vi "- VI Tree - JKI SMO.vi"() -> ()   [LabVIEW 2013, in "JKI SMO.lvclass"]
uses:
  JKI SMO.lvclass
  Typedefs/PrivateData--Cluster.ctl
  Typedefs/ProtectedEvents--Cluster.ctl
  Typedefs/StopProcessEventData--Cluster.ctl
  Typedefs/AbortProcessEventData--Cluster.ctl
  Typedefs/RegisteredProcessData--Cluster.ctl
panel:
  in  "JKI SMO.lvclass":refnum<class "JKI SMO.lvclass">
  in  "Process Data":T1
  out "Protected Events":T2
  in  "Abort Processes Event Data":T3
  in  "Stop Processes Event Data":T4
  in  "Private Data":T5
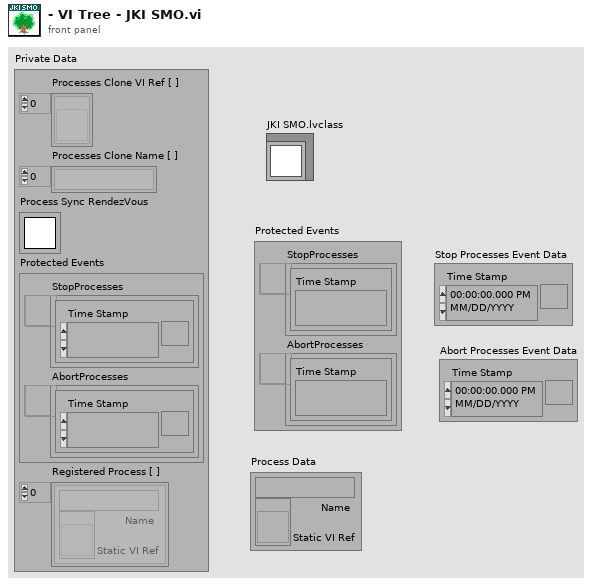
[diagram p1: front panel]
types:
  T1 = typedef "JKI SMO.lvclass/RegisteredProcessData--Cluster.ctl" = cluster{"Name":string, "Static VI Ref":refnum<vi>}
  T2 = typedef "JKI SMO.lvclass/ProtectedEvents--Cluster.ctl" = cluster{"StopProcesses":refnum<user-event>, "AbortProcesses":refnum<user-event>}
  T3 = typedef "JKI SMO.lvclass/AbortProcessEventData--Cluster.ctl" = cluster{"Time Stamp":timestamp}
  T4 = typedef "JKI SMO.lvclass/StopProcessEventData--Cluster.ctl" = cluster{"Time Stamp":timestamp}
  T5 = typedef "JKI SMO.lvclass/PrivateData--Cluster.ctl" = cluster{"Processes Clone VI Ref [ ]":refnum<vi>[], "Processes Clone Name [ ]":string[], "Process Sync RendezVous":T6, "Protected Events":T2, "Registered Process [ ]":T1[]}
  T6 = typedef "Rendezvous RefNum" = refnum<k1>
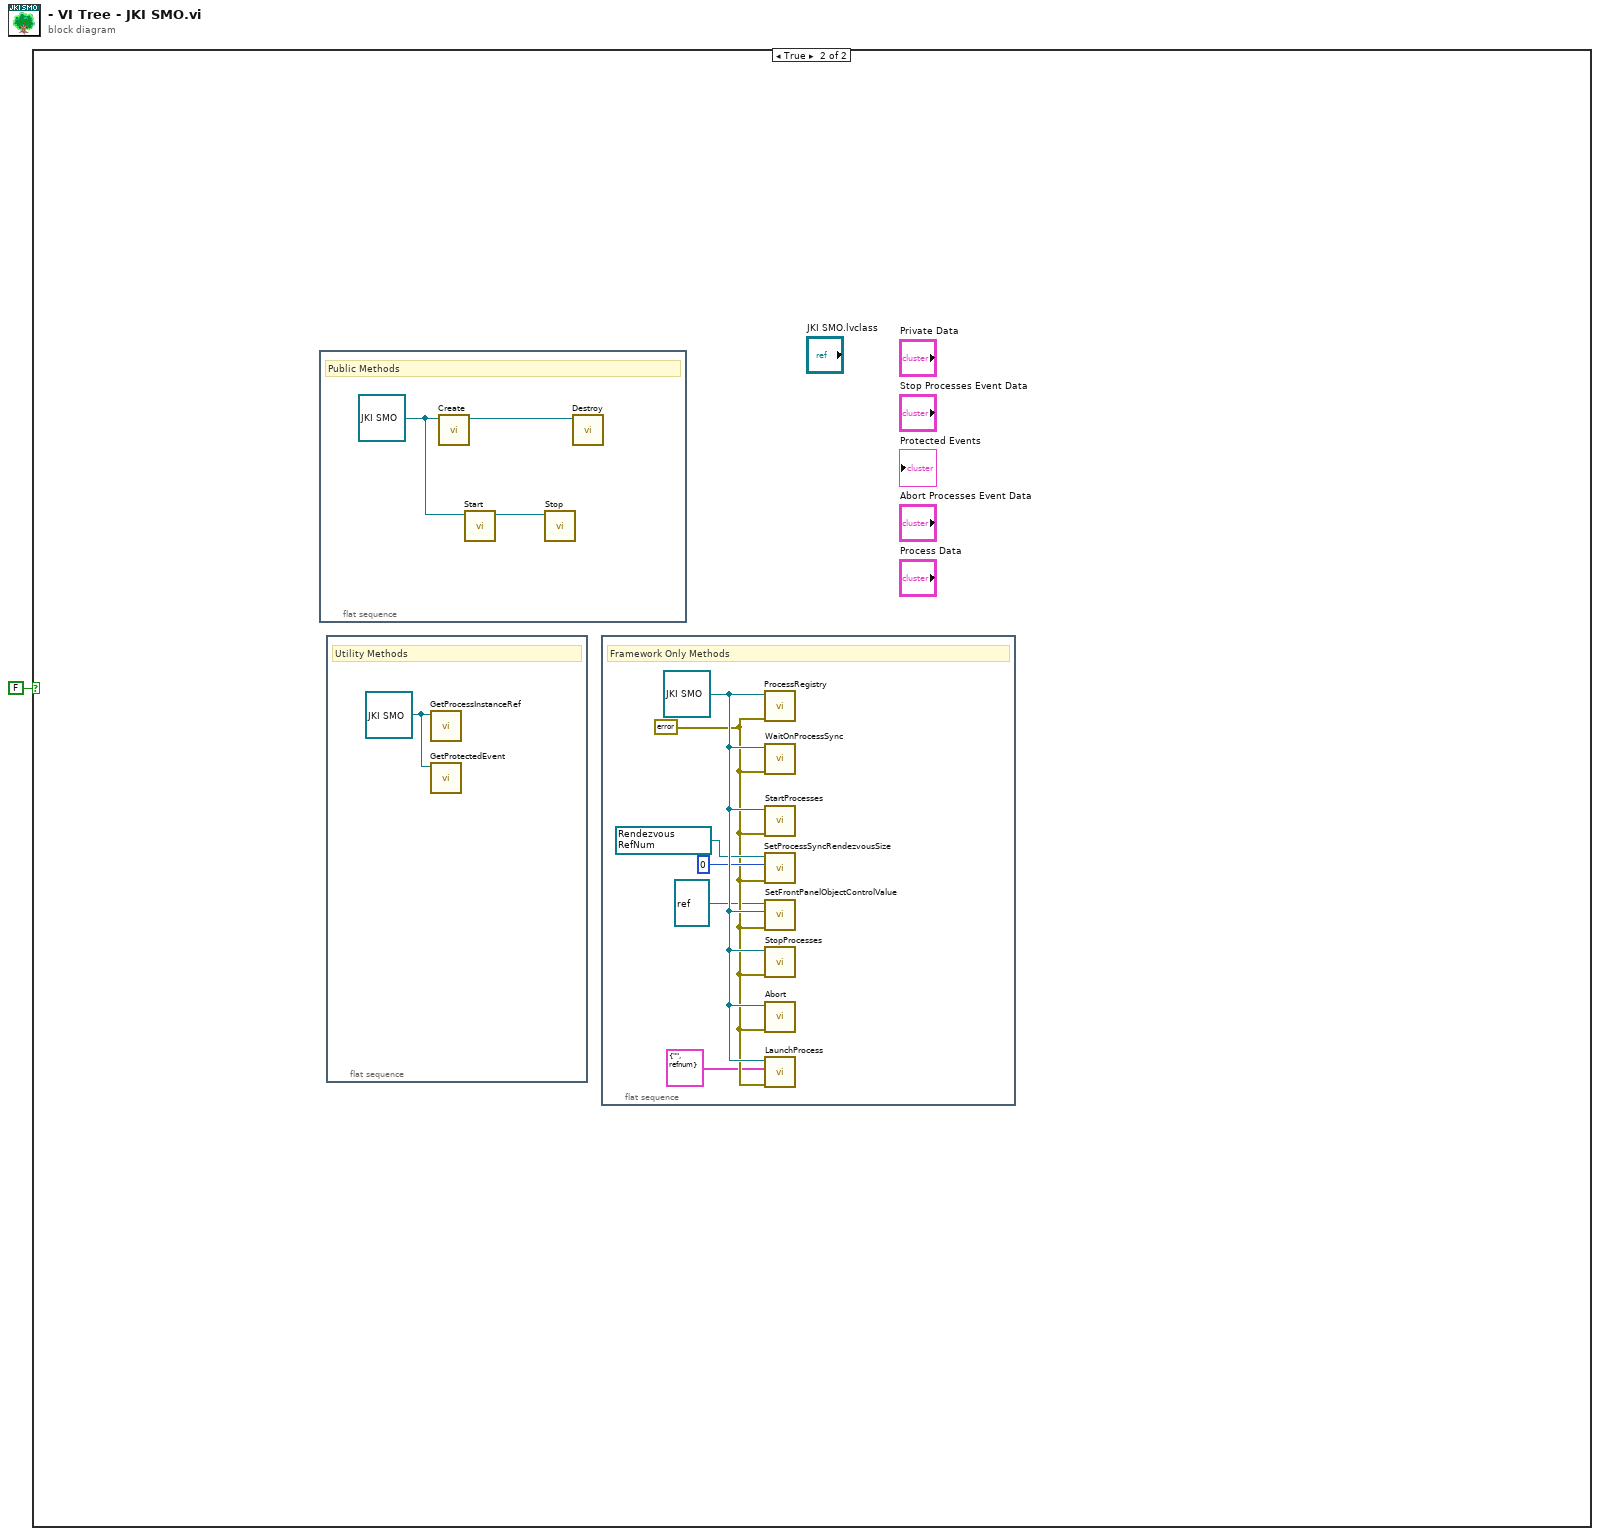
[diagram p0: block diagram]
diagram:
  n1 = case shown="True" FALSE {
    frame False {
    }
    frame True {
      n2 = flat-sequence {
        frame #0 {
          w3 = refnum<class "JKI SMO.lvclass"> refnum ("JKI SMO in")
          # "Public Methods"
          n3 = call-dynamic "Create.vi"("JKI SMO in"=w3) -> ("JKI SMO out"=w4:refnum<class "JKI SMO.lvclass">)  [unwired: 9 in, 1 out]
          n4 = call-dynamic "Start.vi"("JKI SMO in"=w3) -> ("JKI SMO out"=w5:refnum<class "JKI SMO.lvclass">)  [unwired: 9 in, 1 out]
          n5 = call-dynamic "Stop.vi"("JKI SMO in"=w5) -> ()  [unwired: 9 in, 2 out]
          n6 = call-dynamic "Destroy.vi"("JKI SMO in"=w4) -> ()  [unwired: 10 in, 1 out]
        }
      }
      n7 = flat-sequence {
        frame #0 {
          w2 = refnum<class "JKI SMO.lvclass"> refnum ("JKI SMO in")
          # "Utility Methods"
          n8 = call "GetProcessInstanceRef.vi"("JKI SMO in"=w2) -> ()  [unwired: 8 in, 3 out]
          n9 = call "GetProtectedEvent.vi"("JKI SMO in"=w2) -> ()  [unwired: 8 in, 3 out]
        }
      }
      n10 = flat-sequence {
        frame #0 {
          w8 = errorcluster {"status"=FALSE, "code"=0, "source"=""} ("error in")
          w10 = T6 refnum items=["rendezvous"] ("Process Sync Rendezvous")
          w11 = refnum<class "JKI SMO.lvclass"> refnum ("JKI SMO in")
          # "Framework Only Methods"
          n11 = call-dynamic "ProcessRegistry.vi"("error in (no error)"=w8, "pSubSystem in"=w11) -> ()  [unwired: 8 in, 2 out]
          n12 = call "WaitOnProcessSync.vi"("error in (no error)"=w8, "JKI SMO in"=w11) -> ()  [unwired: 8 in, 2 out]
          n13 = call "StartProcesses.vi"("error in (no error)"=w8, "pSubSystem in"=w11) -> ()  [unwired: 8 in, 2 out]
          n14 = call "SetProcessSyncRendezvousSize.vi"("error in"=w8, "# processes"=0, "Process Sync Rendezvous"=w10) -> ()  [unwired: 8 in, 1 out]
          n15 = call "SetFrontPanelObjectControlValue.vi"("error in (no error)"=w8, "JKI SMO in"=w11, "VI Ref In"=refnum<vi> refnum) -> ()  [unwired: 7 in, 2 out]
          n16 = call "StopProcesses.vi"("error in (no error)"=w8, "JKI SMO in"=w11) -> ()  [unwired: 8 in, 2 out]
          n17 = call "Abort.vi"("error in (no error)"=w8, "JKI SMO in"=w11) -> ()  [unwired: 8 in, 2 out]
          n18 = call "LaunchProcess.vi"("error in (no error)"=w8, "Process Data"=T1 {"Name"="", "Static VI Ref"=refnum}, "JKI SMO in"=w11) -> ()  [unwired: 5 in, 4 out]
        }
      }
    }
  }
